vi "Get CmdResp Refs.vi"(8 "error in (no error)":errorcluster, 11 "Section Ref in":T1 format="%.0x") -> (0 "error out":errorcluster, 2 "Signals":T2 {"Cmd Refs" format="%.0x"; "Resp Refs" format="%.0x"}, 3 "Section Ref out":T1 format="%.0x")   [LabVIEW 2015, in "Diagnostics Addon System Explorer.lvlib"]
uses:
  Diagnostics Addon System Explorer.lvlib
  Shared/Types/CmdResp Refs.ctl
  <vilib>/NI Veristand/Custom Device API/Custom Device Item Ref.ctl
  <vilib>/NI Veristand/Custom Device Tools/Custom Device Utility Library/NI VeriStand - Search for Item by GUID.vi
  Shared/SubVIs/GUID Lookup.vi
  <vilib>/NI Veristand/Custom Device API/Custom Device API.lvlib
  <vilib>/NI Veristand/Custom Device Tools/Custom Device Utility Library/Custom Device Utility Library.lvlib
  Shared/Diagnostics Addon Shared.lvlib
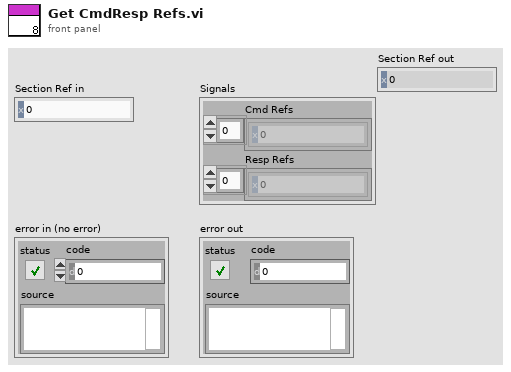
[diagram p1: front panel]
types:
  T1 = typedef "Custom Device API.lvlib/Custom Device Item Ref.ctl" = u64
  T2 = typedef "Diagnostics Addon Shared.lvlib/CmdResp Refs.ctl" = cluster{"Cmd Refs":T1[], "Resp Refs":T1[]}
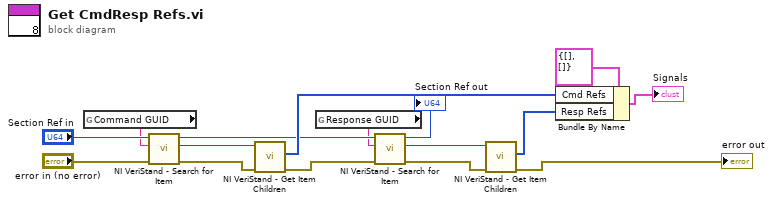
[diagram p0: block diagram]
diagram:
  n1 = global read "GUID Lookup.vi" "Command GUID"() -> (w3:string)
  n2 = call-poly <vilib>:"NI VeriStand - Search for Item.vi"("error in"="error in (no error)", "Item GUID"=w3, "Section Ref in"="Section Ref in") -> ("error out"=w5:errorcluster, "Item Ref"=w4:T1, "Section Ref out"=w6:T1)  [unwired: 5 in, 1 out]
  n3 = call <vilib>:"NI VeriStand - Get Item Children.vi"("error in (no error)"=w5, "Item Ref in"=w4) -> ("error out"=w7:errorcluster, "Child Refs"=w14:T1[])  [unwired: 6 in, 2 out]
  n4 = global read "GUID Lookup.vi" "Response GUID"() -> (w2:string)
  n5 = call-poly <vilib>:"NI VeriStand - Search for Item.vi"("error in"=w7, "Item GUID"=w2, "Section Ref in"=w6) -> ("error out"=w9:errorcluster, "Item Ref"=w8:T1, "Section Ref out"=→"Section Ref out":T1)  [unwired: 5 in, 1 out]
  n6 = call <vilib>:"NI VeriStand - Get Item Children.vi"("error in (no error)"=w9, "Item Ref in"=w8) -> ("error out"=→"error out":errorcluster, "Child Refs"=w15:T1[])  [unwired: 6 in, 2 out]
  n7 = Bundle By Name(cluster=T2 {"Cmd Refs"=[], "Resp Refs"=[]} ("Signals"), "Cmd Refs"=w14, "Resp Refs"=w15) -> (→"Signals":T2)
